vi "up_grid_data_freq.vi"(9 "Data.V_Downstream":T1, 10 "Data.V_UpStream":T1) -> (0 "ctrl var":dbl, 1 "reference":dbl, 2 "upper layer grid info":T3)   [LabVIEW 2021]
uses:
  3ph Phasor.ctl
  Phasor.ctl
  <vilib>/Analysis/baseanly.llb/Mean (DBL).vi
  <vilib>/Analysis/baseanly.llb/Complex A x Vector.vi
  <vilib>/Analysis/Matrix/Numeric/Conversions/Array To Matrix - CA2.vi
  <vilib>/Analysis/NI_AALBase.lvlib
  <vilib>/Analysis/Matrix/NI_Matrix.lvlib
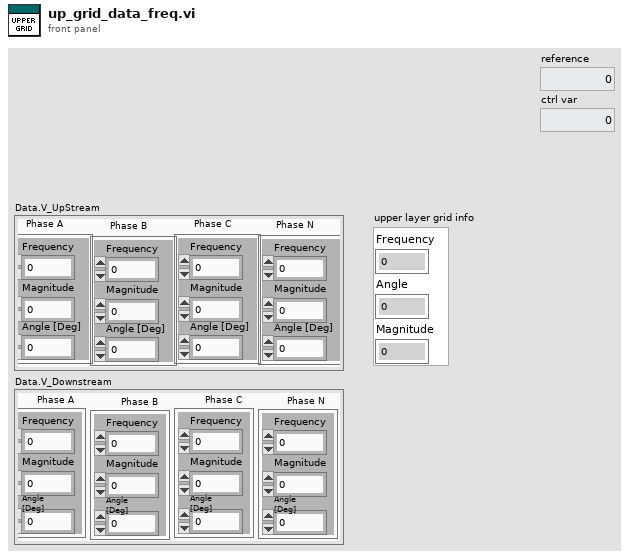
[diagram p1: front panel]
types:
  T1 = typedef "3ph Phasor.ctl" = cluster{"Phase A":T2, "Phase B":T2, "Phase C":T2, "Phase N":T2}
  T2 = typedef "Phasor.ctl" = cluster{"Frequency":dbl, "Magnitude":dbl, "Angle [Deg]":dbl}
  T3 = cluster{"Frequency":dbl, "Angle":dbl, "Magnitude":dbl}
  T4 = typedef "NI_Matrix.lvlib/ComplexMatrix.ctl" = cdb[][]
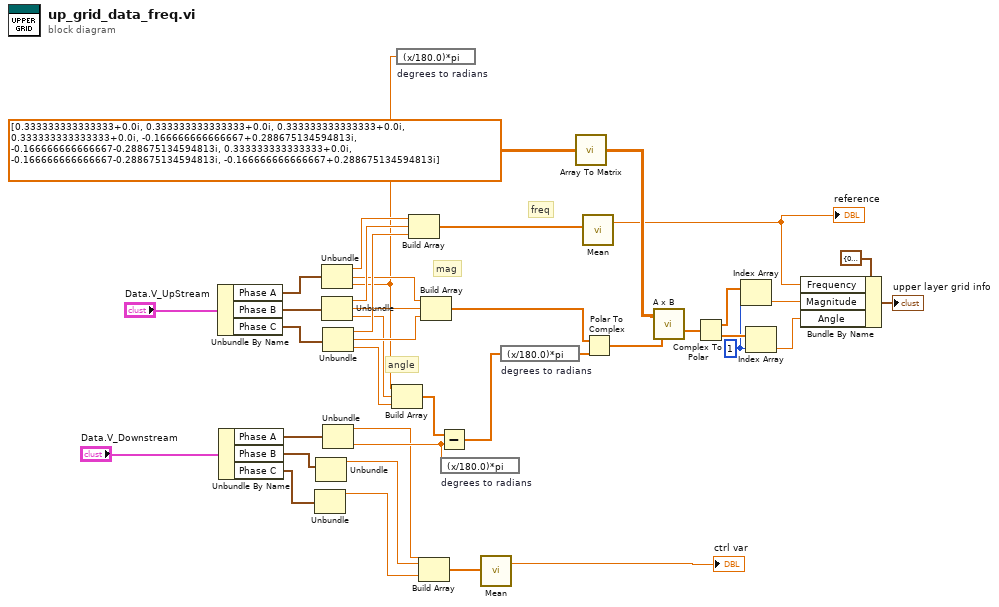
[diagram p0: block diagram]
diagram:
  w20 = 1 ("index")
  # "angle"
  # "mag"
  # "freq"
  n1 = Unbundle By Name("Data.V_UpStream") -> ("Phase A"=w37:T2, "Phase B"=w36:T2, "Phase C"=w35:T2)
  n2 = Unbundle By Name("Data.V_Downstream") -> ("Phase A"=w19:T2, "Phase B"=w8:T2, "Phase C"=w7:T2)
  n3 = Unbundle(w7) -> ("Frequency"=w4:dbl)  [unwired: 2 out]
  n4 = Unbundle(w8) -> ("Frequency"=w5:dbl)  [unwired: 2 out]
  n5 = Unbundle(w37) -> ("Frequency"=w34:dbl, "Magnitude"=w31:dbl, "Angle [Deg]"=w10:dbl)
  n6 = Unbundle(w36) -> ("Frequency"=w33:dbl, "Magnitude"=w30:dbl, "Angle [Deg]"=w28:dbl)
  n7 = Unbundle(w35) -> ("Frequency"=w32:dbl, "Magnitude"=w29:dbl, "Angle [Deg]"=w27:dbl)
  n8 = Unbundle(w19) -> ("Frequency"=w6:dbl, "Angle [Deg]"=w9:dbl)  [unwired: 1 out]
  n9 = Build Array(w10, w28, w27) -> (w11:dbl[])
  n10 = expression code="(x/180.0)*pi" "degrees to radians"(w10) -> ()  [unwired: 1 out]
  n11 = Build Array(w34, w33, w32) -> (w26:dbl[])
  n12 = Build Array(w6, w5, w4) -> (w3:dbl[])
  n13 = Build Array(w31, w30, w29) -> (w25:dbl[])
  n14 = Subtract(x=w11, y=w9) -> (x-y=w12:dbl[])
  n15 = expression code="(x/180.0)*pi" "degrees to radians"(w9) -> ()  [unwired: 1 out]
  n16 = call-poly <vilib>:"Mean.vi"("X"=w3) -> ("mean"=→"ctrl var":dbl)  [unwired: 1 out]
  n17 = expression code="(x/180.0)*pi" "degrees to radians"(w12) -> (w13:dbl[])
  n18 = call-poly <vilib>:"Array To Matrix.vi"("Complex 2D Array"=cdb[][] [[0.333333333333333+0.0i, 0.333333333333333+0.0i, 0.333333333333333+0.0i], [0.333333333333333+0.0i, -0.166666666666667+0.288675134594813i, -0.166666666666667-0.288675134594813i], [0.333333333333333+0.0i, -0.166666666666667-0.288675134594813i, -0.166666666666667+0.288675134594813i]] ("r * e^(i*theta)")) -> ("Complex Matrix"=w14:T4)
  n19 = call-poly <vilib>:"Mean.vi"("X"=w26) -> ("mean"=w2:dbl)  [unwired: 1 out]
  "reference" <- w2
  n20 = Polar To Complex(1:w13, 2:w25) -> (0:w17:cdb[])
  n21 = call-poly <vilib>:"A x B.vi"("Vector"=w17, "A"=w14) -> ("A x Vector"=w16:cdb[])  [unwired: 1 out]
  n22 = Complex To Polar ("Complex To Polar.vi")(r * e^(i*theta)=w16) -> (r=w23:dbl[], theta=w21:dbl[])
  n23 = Index Array(array=w23, index=w20) -> (element=w24:dbl)
  n24 = Index Array(array=w21, index=w20) -> (element=w22:dbl)
  n25 = Bundle By Name(cluster=T3 {"Frequency"=0.0, "Angle"=0.0, "Magnitude"=0.0} ("upper layer grid info"), "Frequency"=w2, "Magnitude"=w24, "Angle"=w22) -> (→"upper layer grid info":T3)
